vi "Write Control Limits - Low Limit.vi"(8 "error in (no error)":errorcluster, 10 "low limit":dbl, 11 "NT Scalar (Numeric) in":refnum<class "NT Scalar (Numeric).lvclass">) -> (0 "error out":errorcluster, 3 "NT Scalar (Numeric) out":refnum<class "NT Scalar (Numeric).lvclass">)   [LabVIEW 2020, in "PV Access.lvlib" / "PV Data.lvlib" / "NT Scalar (Numeric).lvclass"]
uses:
  NT Scalar (Numeric).lvclass
  NT Scalar (Numeric).lvclass/NT Scalar (Numeric).ctl
  8f228ecd-0a3d-4825-8ae7-6ec3fb9e8929.vi
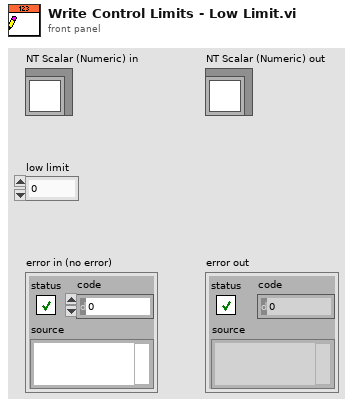
[diagram p1: front panel]
types:
  T1 = typedef "PV Access.lvlib/PV Data.lvlib/Type Code.ctl" = enum8{"Null", "Bool", "BoolA", "Int8", "Int8A", "Int16", "Int16A", "Int32", "Int32A", "Int64", "Int64A", "UInt8", "UInt8A", "UInt16", "UInt16A", "UInt32", "UInt32A", "UInt64", "UInt64A", "Float32", "Float32A", "Float64", "Float64A", "String", "StringA", "Struct", "StructA", "Union", "UnionA", "Any", "AnyA"}
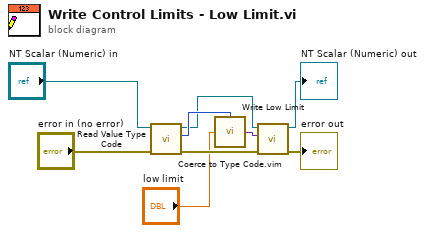
[diagram p0: block diagram]
diagram:
  n1 = call-dynamic "Read Value Type Code.vi"("error in (no error)"="error in (no error)", "NT Scalar in"="NT Scalar (Numeric) in") -> ("error out"=w5:errorcluster, "type code"=w7:T1, "NT Scalar out"=w3:refnum<class "NT Scalar (Numeric).lvclass">)  [unwired: 7 in]
  n2 = call "Coerce to Type Code.vim"("type code"=w7, "value in"="low limit") -> ("value out"=w1:variant)  [unwired: 2 in]
  n3 = call-dynamic "Write Low Limit.vi"("error in"=w5, "low limit"=w1, "Has Control Limits in"=w3) -> ("error out"=→"error out":errorcluster, "Has Control Limits out"=→"NT Scalar (Numeric) out":refnum<class "NT Scalar (Numeric).lvclass">)  [unwired: 7 in]
